vi "path.vi"() -> (0 "lib path":path)   [LabVIEW 2019, in "D2XX.lvlib"]
uses:
  D2XX.lvlib
  i386/i386.lvclass
  amd64/amd64.lvclass
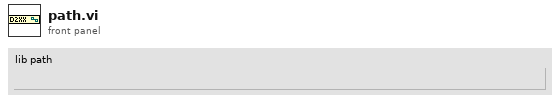
[diagram p1: front panel]
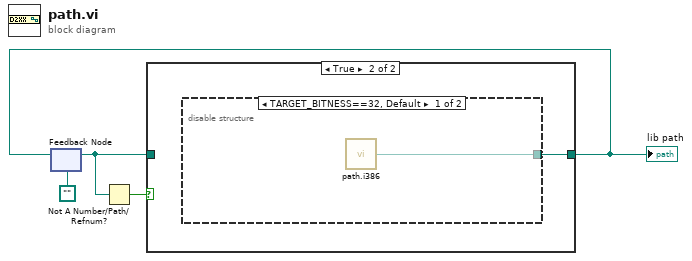
[diagram p0: block diagram]
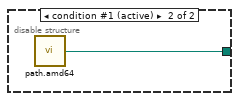
[diagram p3: hidden frame]
diagram:
  n1 = feedback #1(path "") -> (w2:path)
  n2 = Not A Number/Path/Refnum?(number/path/refnum=w2) -> (NaN/Path/Refnum?=w3:bool)
  n3 = case shown="True" w3 {
    tunnel: [w5 w6] -> w1
    tunnel: w2 -> [w5 _]
    frame False {
    }
    frame True {
      n4 = disable-structure shown="TARGET_BITNESS==32, Default" {
        disable-tunnel: [w7 w8] -> w6
        frame condition #0 {
          n5 = call "path.i386.vi"() -> ("lib path"=w7:path)
        }
        frame condition #1 (active) {
          n6 = call "path.amd64.vi"() -> ("lib path"=w8:path)
        }
      }
    }
  }
  "lib path" <- w1
  n7 = feedback-in #1(w1) -> ()
